vi "WLM Wait event.vi"(8 "error in (no error)":errorcluster, 10 "wait event":enum16{"install", "remove"}(ring)) -> (0 "error out":errorcluster, 2 "return value":u32)   [LabVIEW 2009]
doc: "Installs or removes a wait event, which is necessary before checking for changes in the WLM."
uses:
  <vilib>/Utility/error.llb/DialogType.ctl
  WINDOWS/system32/wlmData.dll
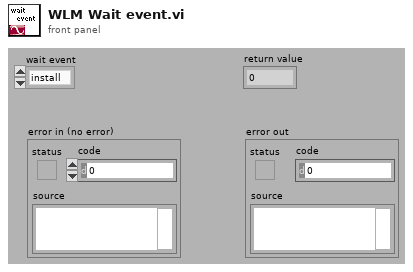
[diagram p1: front panel]
types:
  T1 = typedef "DialogType.ctl" = u16
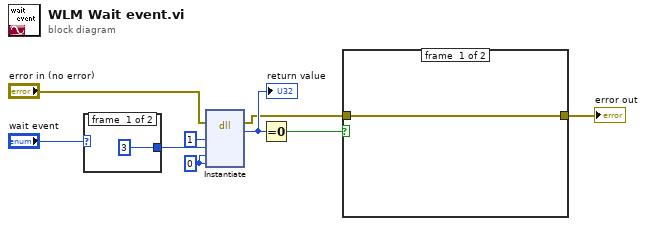
[diagram p0: block diagram]
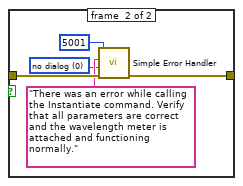
[diagram p2: hidden frame]
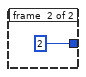
[diagram p3: hidden frame]
diagram:
  w9 = u32 0 ("P2")
  n1 = case shown="\"install\", Default" "wait event" {
    tunnel: [u32 3 u32 2] -> w6
    frame #0 {
    }
    frame #1 {
    }
  }
  n2 = dll-call lib="C:/WINDOWS/system32/wlmData.dll" fn="Instantiate"(error in="error in (no error)", "RFC"=u32 1, "Mode"=w6, "P1"=w9, "P2"=w9) -> (error out=w2:errorcluster, "return type"=w3:u32)  [unwired: 6 in, 1 out]
  "return value" <- w3
  n3 = Equal To 0?(x=w3) -> (x = 0?=w4:bool)
  n4 = case shown="True" w4 {
    tunnel: w2 -> [w12 w17]
    tunnel: [w12 w14] -> w1
    frame #0 {
    }
    frame #1 {
      w15 = T1 0 items=["no dialog", "OK message", "continue or stop message", "OK message + warnings", "continue/stop + warnings"] ("type of dialog (OK msg:1)")
      n5 = call <vilib>:"Simple Error Handler.vi"("error code (no error:0)"=5001, "error source (\" \")"="There was an error while calling the Instantiate command. Verify that all parameters are correct and the wavelength meter is attached and functioning normally." ("error source (\" \")"), "type of dialog (OK msg:1)"=w15, "error in (no error)"=w17) -> ("error out"=w14:errorcluster)  [unwired: 5 out]
    }
  }
  "error out" <- w1
